vi "NT IsConnected.vi"() -> (0 "Error":errorcluster={"status"=FALSE, "code"=-1, "source"=""}, 3 "Connected":bool)   [LabVIEW 2019, in "Trajectory_Library.lvlib"]
doc: "Returns TRUE if connected to an NT Server. This can be called periodically to determine if a valid NT server connection exists.\n\nInputs:\n - <none>\n\nOutputs:\n - Connected - boolean - Returns TRUE if a valid NT server connection exists."
uses:
  Trajectory_Library.lvlib
  ntcoreffi.dll
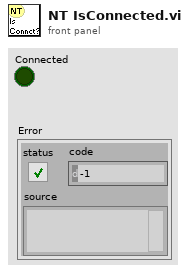
[diagram p1: front panel]
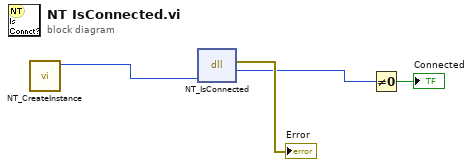
[diagram p0: block diagram]
diagram:
  n1 = call <vilib>:"NT_CreateInstance.vi"() -> ("InstanceHandle"=w3:u64)  [unwired: 10 in, 1 out]
  n2 = dll-call lib="ntcoreffi.*" fn="NT_IsConnected"("inst"=w3) -> (error out=→"Error":errorcluster, "return type"=w2:u32)  [unwired: 4 in, 1 out]
  n3 = Not Equal To 0?(x=w2) -> (x != 0?=→"Connected":bool)
